vi "Pockels-Initial checks prompt.vi"(8 "error in (no error)":errorcluster) -> (0 "error out":errorcluster)   [LabVIEW 2017]
uses:
  Typedefs/Functional global standard states.ctl
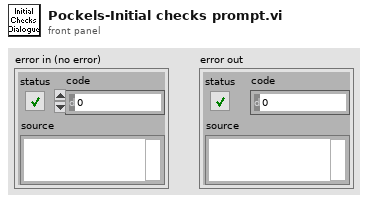
[diagram p1: front panel]
types:
  T1 = typedef "Functional global standard states.ctl" = enum16{"Initialise", "Read", "Write", "Load", "Save", "Clear"}
  T2 = typedef "Pockels cal conditions cluster.ctl" = cluster{"Wavelength":u16, "Zoom":u8, "Dwell time (us)":dbl, "Pockels bias":i16, "Prism 1":u16, "Prism 2":u16, "Laser power during pockels cal (mW)":u16}
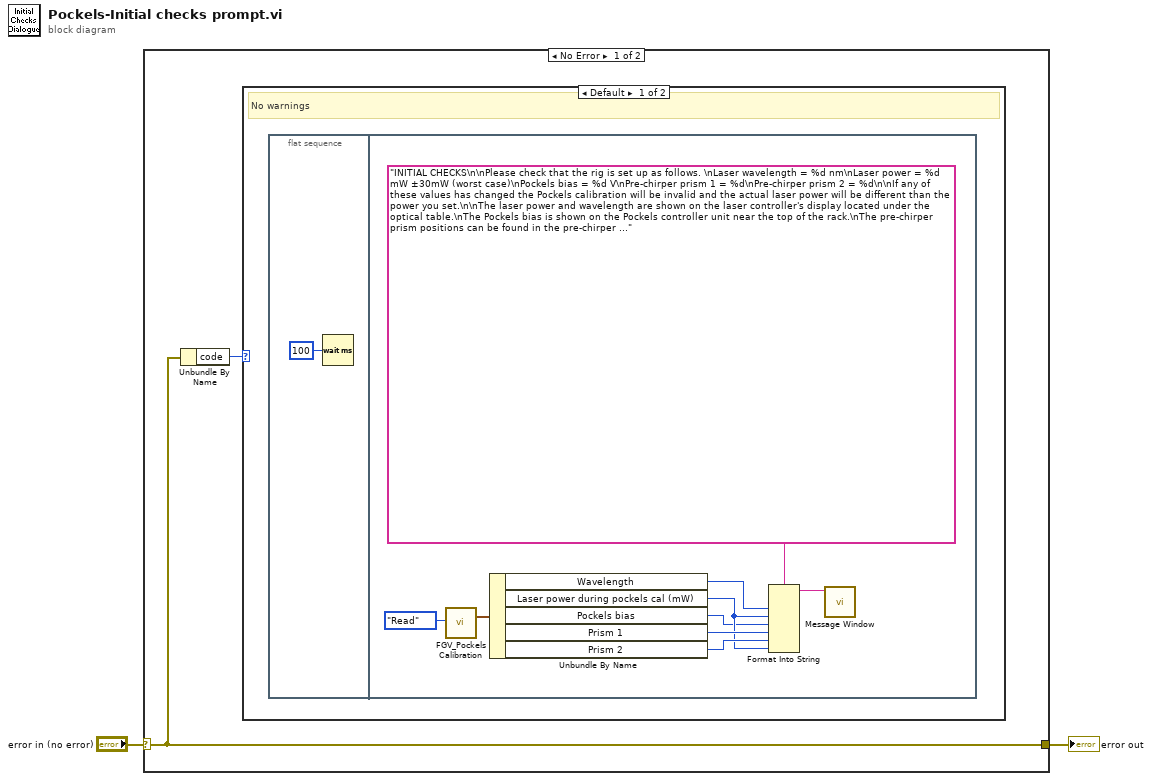
[diagram p0: block diagram]
diagram:
  n1 = case shown="No Error" "error in (no error)" {
    selector: "error in (no error)" -> [w4 w15]
    tunnel: [w4 w15] -> w1
    frame No Error {
      n2 = Unbundle By Name(w4) -> ("code"=w3:i32)
      n3 = case shown="Default" w3 {
        frame Default {
          # "No warnings"
          n4 = flat-sequence {
            frame #0 {
              n5 = Wait (ms)(milliseconds to wait=u32 100) -> ()  [unwired: 1 out]
            }
            frame #1 {
              n6 = call "FGV_Pockels Calibration.vi"("Function"=Functional_global_standard_states."Read") -> ("Cal conditions"=w12:T2)  [unwired: 4 in, 6 out]
              n7 = Unbundle By Name(w12) -> ("Wavelength"=w6:u16, "Laser power during pockels cal (mW)"=w8:u16, "Pockels bias"=w7:i16, "Prism 1"=w10:u16, "Prism 2"=w9:u16)
              n8 = Format Into String(format string="INITIAL CHECKS\n\nPlease check that the rig is set up as follows. \nLaser wavelength = %d nm\nLaser power = %d mW ±30mW (worst case)\nPockels bias = %d V\nPre-chirper prism 1 = %d\nPre-chirper prism 2 = %d\n\nIf any of these values has changed the Pockels calibration will be invalid and the actual laser power will be different than the power you set.\n\nThe laser power and wavelength are shown on the laser controller's display located under the optical table.\nThe Pockels bias is shown on the Pockels controller unit near the top of the rack.\nThe pre-chirper prism positions can be found in the pre-chirper control unit in the rack.\n\nNote that it takes approximately an hour for the laser controller to stabilise. If the value shown on the controller is not %dmW you can try allowing some extra time for the controller to stabilise.\n\nIf the discrepancy persists, in most cases this means something has changed in the optics setup, in which case the Pockels will need to be recalibrated before experiments can commence.\n\nPockels calibration is carried out using the relevant wizard available through the Config menu.\nConfig>Calibration>Pockels calibration wizard\n" ("Message string"), w6, w8, w7, w10, w9, w8) -> (resulting string=w11:string)  [unwired: 2 in, 1 out]
              n9 = call "Message Window.vi"("Message string"=w11) -> ()  [unwired: 10 in, 1 out]
            }
          }
        }
        frame 5003..5005 {
          # "Pockels cal warnings / Default cal has been loaded"
        }
      }
    }
    frame Error {
    }
  }
  "error out" <- w1
